vi "Serial fit Lc, Lp and K.vi"(0 "Extension (nm)":dbl[](array[numeric]), 2 "Force (pN)":dbl[](array[numeric]), 5 "initial parameters for eWLC (Lc,Lp,K)":dbl[](array[numeric])=[1000.0, 1200.0]) -> (4 "Cut-Force (pN)":dbl[](array[numeric]), 6 "best fit parameters for eWLC":dbl[](array[numeric]), 8 "best nonlinear fit for eWLC":dbl[](array[numeric]))   [LabVIEW 2014]
uses:
  <vilib>/gmath/NumericalOptimization/Nonlinear Curve Fit LM formula string.vi
  <vilib>/gmath/NI_Gmath.lvlib
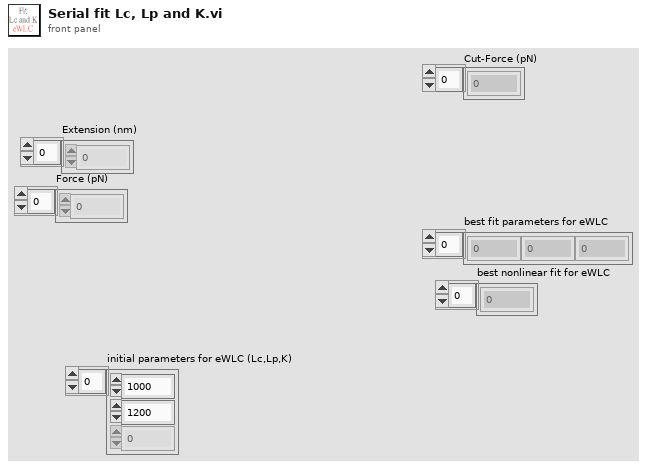
[diagram p1: front panel]
types:
  T1 = cluster{"model":string, "Parameters":string[], "x":string}
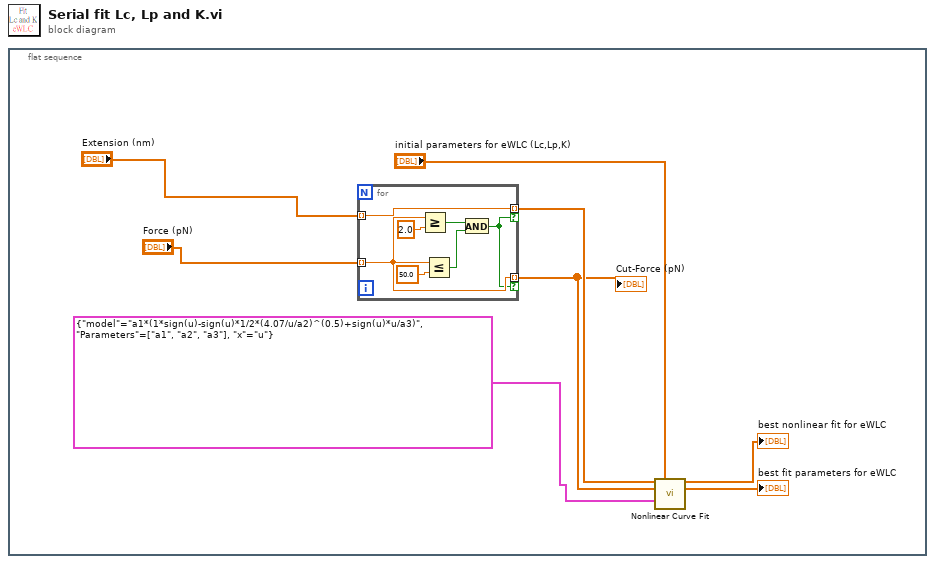
[diagram p0: block diagram]
diagram:
  n1 = flat-sequence {
    frame #0 {
      n2 = for {
        tunnel: "Force (pN)" -> [w13] mode=indexing
        tunnel: [w13] -> w4 mode=indexing if=w9
        tunnel: "Extension (nm)" -> [w14] mode=indexing
        tunnel: [w14] -> w5 mode=indexing if=w9
        n3 = Greater Or Equal?(x=w13, y=2.0) -> (x >= y?=w11:bool)
        n4 = Less Or Equal?(x=w13, y=50.0) -> (x <= y?=w10:bool)
        n5 = And(x=w11, y=w10) -> (x .and. y?=w9:bool)
      }
      "Cut-Force (pN)" <- w4
      n6 = call-poly <vilib>:"Nonlinear Curve Fit.vi"("Y"=w5, "initial parameters"="initial parameters for eWLC (Lc,Lp,K)", "X"=w4, "model description"=T1 {"model"="a1*(1*sign(u)-sign(u)*1/2*(4.07/u/a2)^(0.5)+sign(u)*u/a3)", "Parameters"=["a1", "a2", "a3"], "x"="u"}) -> ("best nonlinear fit"=→"best nonlinear fit for eWLC":dbl[], "best fit parameters"=→"best fit parameters for eWLC":dbl[])  [unwired: 3 in, 7 out]
    }
  }
